vi "List Folder.vi"(8 "error in (no error)":errorcluster, 10 "folder (root)":string, 11 "Artifactory in":refnum<class "Artifactory.lvclass">) -> (0 "error out":errorcluster, 1 "Files":string[](array[string]), 2 "Folders":string[](array[string]), 3 "Artifactory out":refnum<class "Artifactory.lvclass">)   [LabVIEW 2021, in "Artifactory.lvclass"]
uses:
  Artifactory.lvclass
  <vilib>/LabVIEW Open Source Project/OpenURI/uri/URI.lvclass
  Artifactory.lvclass/Artifactory.ctl
  <vilib>/LabVIEW Open Source Project/OpenURI/uri/URI.lvclass/URI.ctl
  58a193ed-304a-485f-a0b0-94bd1b85ef9b.vi
  a50ec5f8-b0a9-4898-9a17-bb99d391555f.vi
  f1812c00-ec24-49ff-831b-cd8a90229306.vi
  <vilib>/JDP Science/JSONtext/String Subset.vi
  <vilib>/LabVIEW Open Source Project/OpenURI/components/path/Get path (absolute).vi
  <vilib>/JDP Science/JSONtext/Parsing/Parse Full Path or Item Name.vi
  <vilib>/JDP Science/JSONtext/Next JSON Value.vi
  <vilib>/JDP Science/JSONtext/support/Error Cluster From Code.vi
  <vilib>/JDP Science/JSONtext/Offset/Find Item Locations by Path.vi
  <vilib>/JDP Science/JSONtext/JSON text to Variant.vi
  <vilib>/JDP Science/JSONtext/LVClass Serializer/JSONtext LVClass Serializer.lvclass
  <vilib>/regexp/Match Regular Expression.xnode
  <vilib>/addons/_JKI.lib/REST Client/classes/REST Client/REST Client.lvclass
  <vilib>/JDP Science/JSONtext/JSONtext.lvlib
  Actions -- enum.ctl
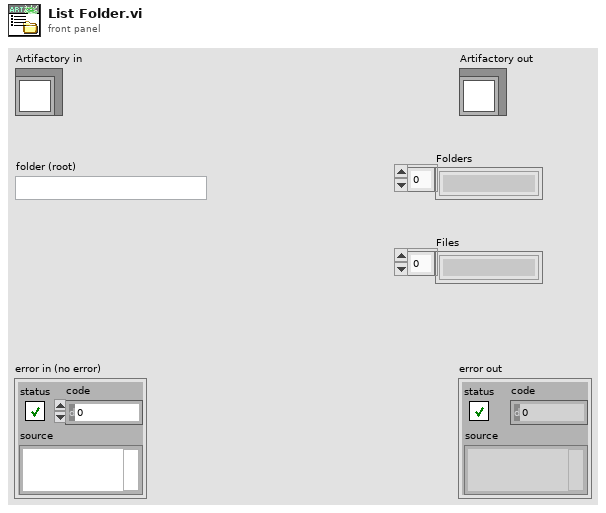
[diagram p1: front panel]
types:
  T1 = typedef "Artifactory.lvclass/Actions -- enum.ctl" = enum16{"Idle", "Custom Event", "Connecting to Artifactory", "Verifying Permissions", "Listing local repository", "Listing remote repository", "Computing changes", "Uploading file", "Downloading file"}
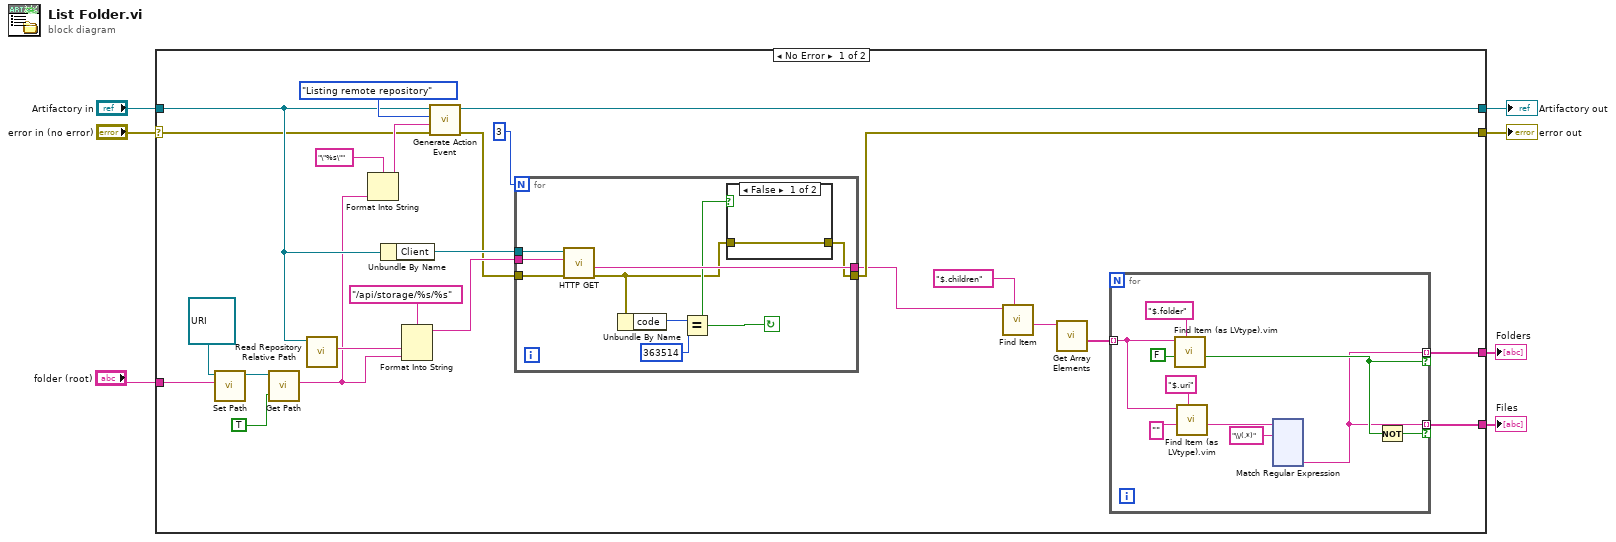
[diagram p0: block diagram]
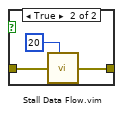
[diagram p2: hidden frame]
diagram:
  n1 = case shown="No Error" "error in (no error)" {
    selector: "error in (no error)" -> [w9 w175]
    tunnel: [w24 w175] -> w6
    tunnel: [w13 w174] -> w4
    tunnel: "Artifactory in" -> [w12 w174]
    tunnel: "folder (root)" -> [w28 _]
    tunnel: [w19 _] -> w2
    tunnel: [w18 _] -> w1
    frame No Error {
      n2 = call <vilib>:"Set Path.vi"("path"=w28, "URI in"=refnum<class "URI.lvclass"> refnum) -> ("URI out"=w26:refnum<class "URI.lvclass">)  [unwired: 8 in, 1 out]
      n3 = call <vilib>:"Get Path.vi"("Strip lead \"/\" (F)"=TRUE ("Strip lead \"/\" (F)"), "URI in"=w26) -> ("path"=w11:string)  [unwired: 7 in, 2 out]
      n4 = call "Read Repository Relative Path.vi"("Artifactory in"=w12) -> ("repository path"=w16:string)  [unwired: 9 in, 1 out]
      n5 = Format Into String(format string="\"%s\"", w11) -> (resulting string=w10:string)  [unwired: 2 in, 1 out]
      n6 = Unbundle By Name(w12) -> ("Client"=w31:refnum<class "REST Client.lvclass">)
      n7 = Format Into String(format string="/api/storage/%s/%s" ("Path"), w16, w11) -> (resulting string=w29:string)  [unwired: 2 in, 1 out]
      n8 = call-dynamic "Generate Action Event.vi"("error in (no error)"=w9, "Description"=w10, "Action"=Actions_--_enum."Listing remote repository", "Artifactory in"=w12) -> ("error out"=w8:errorcluster, "Artifactory out"=w13:refnum<class "Artifactory.lvclass">)  [unwired: 6 in]
      n9 = for {
        N: 3 -> [_]
        tunnel: w31 -> [w40]
        tunnel: w8 -> [w38]
        tunnel: [w32] -> w24
        tunnel: w29 -> [w39]
        tunnel: [w37] -> w21
        stop <- w34 continue-if-true
        n10 = call-dynamic "HTTP GET.vi"("error in (no error)"=w38, "Path"=w39, "REST Client in"=w40) -> ("error out"=w33:errorcluster, "Response body"=w37:string)  [unwired: 3 in, 4 out]
        n11 = Unbundle By Name(w33) -> ("code"=w36:i32)
        n12 = Equal?(x=w36, y=363514) -> (x = y?=w34:bool)
        n13 = case shown="False" w34 {
          tunnel: w33 -> [w41 w44]
          tunnel: [w41 w43] -> w32
          frame False {
          }
          frame True {
            n14 = call "Stall Data Flow.vim"("value in"=w44, "milliseconds to wait"=u32 20) -> ("value out"=w43:errorcluster)  [unwired: 1 out]
          }
        }
      }
      n15 = call <vilib>:"Find Item.vi"("$Path or Item Name"="$.children", "JSON"=w21) -> ("<JSON>"=w22:string)  [unwired: 6 in, 3 out]
      n16 = call <vilib>:"Get Array Elements.vi"("JSON"=w22) -> ("<JSON>"=w20:string[])  [unwired: 8 in, 2 out]
      n17 = for {
        tunnel: w20 -> [w52] mode=indexing
        tunnel: [w45] -> w18 mode=indexing if=w48
        tunnel: [w45] -> w19 mode=indexing if=w49
        n18 = call "Find Item (as LVtype).vim"("$Path or Item Name"="$.folder", "Data Type and Default Value"=FALSE, "JSON"=w52) -> ("Data"=w49:bool)  [unwired: 5 in, 3 out]
        n19 = call "Find Item (as LVtype).vim"("$Path or Item Name"="$.uri", "Data Type and Default Value"="" ("$Path or Item Name"), "JSON"=w52) -> ("Data"=w46:string)  [unwired: 5 in, 3 out]
        n20 = xnode "Match Regular Expression"("input string"=w46, "regular expression"="\\/(.*)") -> ("submatch 1"=w45:string)  [unwired: 4 in, 5 out]
        n21 = Not(x=w49) -> (.not. x?=w48:bool)
      }
    }
    frame Error {
    }
  }
  "error out" <- w6
  "Artifactory out" <- w4
  "Folders" <- w2
  "Files" <- w1
